vi "GetText.vi"(8 "error in":errorcluster, 11 "cRIO in":refnum<class "cRIO.lvclass">) -> (0 "error out":errorcluster, 1 "additional text":string, 2 "text":string, 3 "cRIO out":refnum<class "cRIO.lvclass">, 4 "glyph":string)   [LabVIEW 2013, in "cRIO.lvclass"]
uses:
  cRIO.lvclass
  cRIO.lvclass/cRIO.ctl
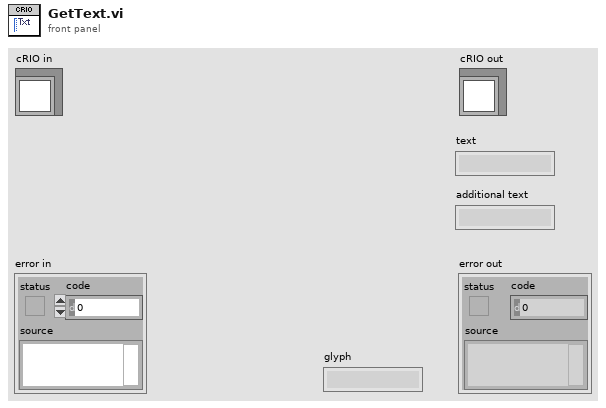
[diagram p1: front panel]
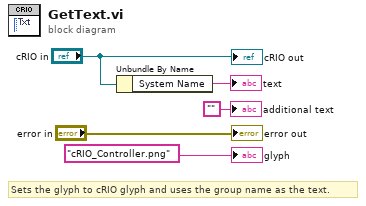
[diagram p0: block diagram]
diagram:
  # "Sets the glyph to cRIO glyph and uses the group name as the text."
  n1 = Unbundle By Name("cRIO in") -> ("System Name"=→"text":string)
  "error out" <- "error in"
  "cRIO out" <- "cRIO in"
  "additional text" <- ""
  "glyph" <- "cRIO_Controller.png" ("glyph")
